vi "ad get digital line.vi"(7 "data":u32, 8 "error in (no error)":errorcluster, 9 "line":i32, 10 "cha":i32, 11 "adh":i32) -> (0 "error out":errorcluster, 3 "function return":i32, 5 "data out":u32)   [LabVIEW 2021, in "libad4.lvlib"]
doc: "LIBAD4 function: ad_get_digital_line (int32_t adh, int32_t cha, int32_t line, uint32_t *data);\n\nGets digital line status."
uses:
  <userlib>/libad4/libad4.lvlib
  <userlib>/libad4/libad4.dll
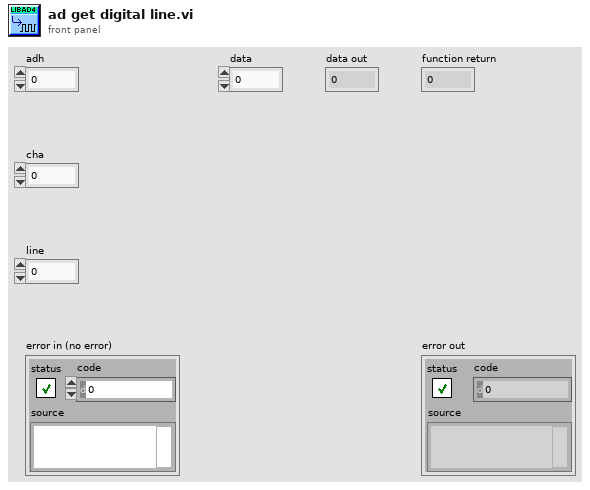
[diagram p1: front panel]
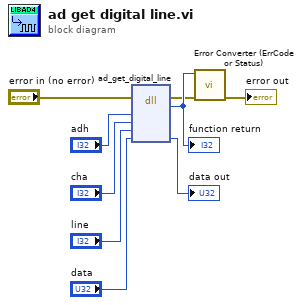
[diagram p0: block diagram]
diagram:
  n1 = dll-call lib="C:/Program Files/National Instruments/LabVIEW 2021/user.lib/libad4/libad4.*" fn="ad_get_digital_line"(error in="error in (no error)", "adh"="adh", "cha"="cha", "line"="line", "data"="data") -> (error out=w2:errorcluster, w9:i32, "data"=→"data out":u32)  [unwired: 5 in, 1 out]
  "function return" <- w9
  n2 = call <userlib>:"Error Converter (ErrCode or Status).vi"("error in (no error)"=w2, "error code"=w9) -> ("error out"=→"error out":errorcluster)  [unwired: 9 in]
